vi "CTRE_PigeonIMU_GetAll.vi"(8 "error in (no error)":errorcluster, 11 "PigeonIMUDevRef":T4={"DeviceStatus"={"status"=FALSE, "code"=0, "source"=""}, "Device Number"=0, "Type"=352321536, "Device ID"=0} {"Type" items=["CAN"=352321536, "TalonSRX"=33554432]}) -> (0 "error out":errorcluster, 2 "Get All":T1 {"Calibration"."CurrentMode" items=["BootTareGryoAccel"=0, "Temperature"=1, "Magnetometer12Pt"=2, "Magnetometer360"=3, "Accelerometer"=5]}, 3 "PigeonIMUDevRef":T4={"DeviceStatus"={"status"=FALSE, "code"=0, "source"=""}, "Device Number"=0, "Type"=352321536, "Device ID"=0} {"Type" items=["CAN"=352321536, "TalonSRX"=33554432]})   [LabVIEW 2016]
uses:
  <vilib>/Rock Robotics/WPI/ThirdParty/Sensors/Pigeon IMU/CTRE_PigeonIMU_DeviceRef.ctl
  <vilib>/Rock Robotics/WPI/ThirdParty/Sensors/Pigeon IMU/CTRE_PigeonIMU_ConnectionType.ctl
  <vilib>/Rock Robotics/WPI/ThirdParty/Sensors/Pigeon IMU/CTRE_PigeonIMU_GlobalStatus.ctl
  <vilib>/Rock Robotics/WPI/ThirdParty/Sensors/Pigeon IMU/CTRE_PigeonIMU_PigeonState.ctl
  <vilib>/Rock Robotics/WPI/ThirdParty/Sensors/Pigeon IMU/CTRE_PigeonIMU_CalibrationMode.ctl
  <vilib>/Rock Robotics/WPI/ThirdParty/Sensors/Pigeon IMU/CTRE_PigeonIMU_GlobalOps.ctl
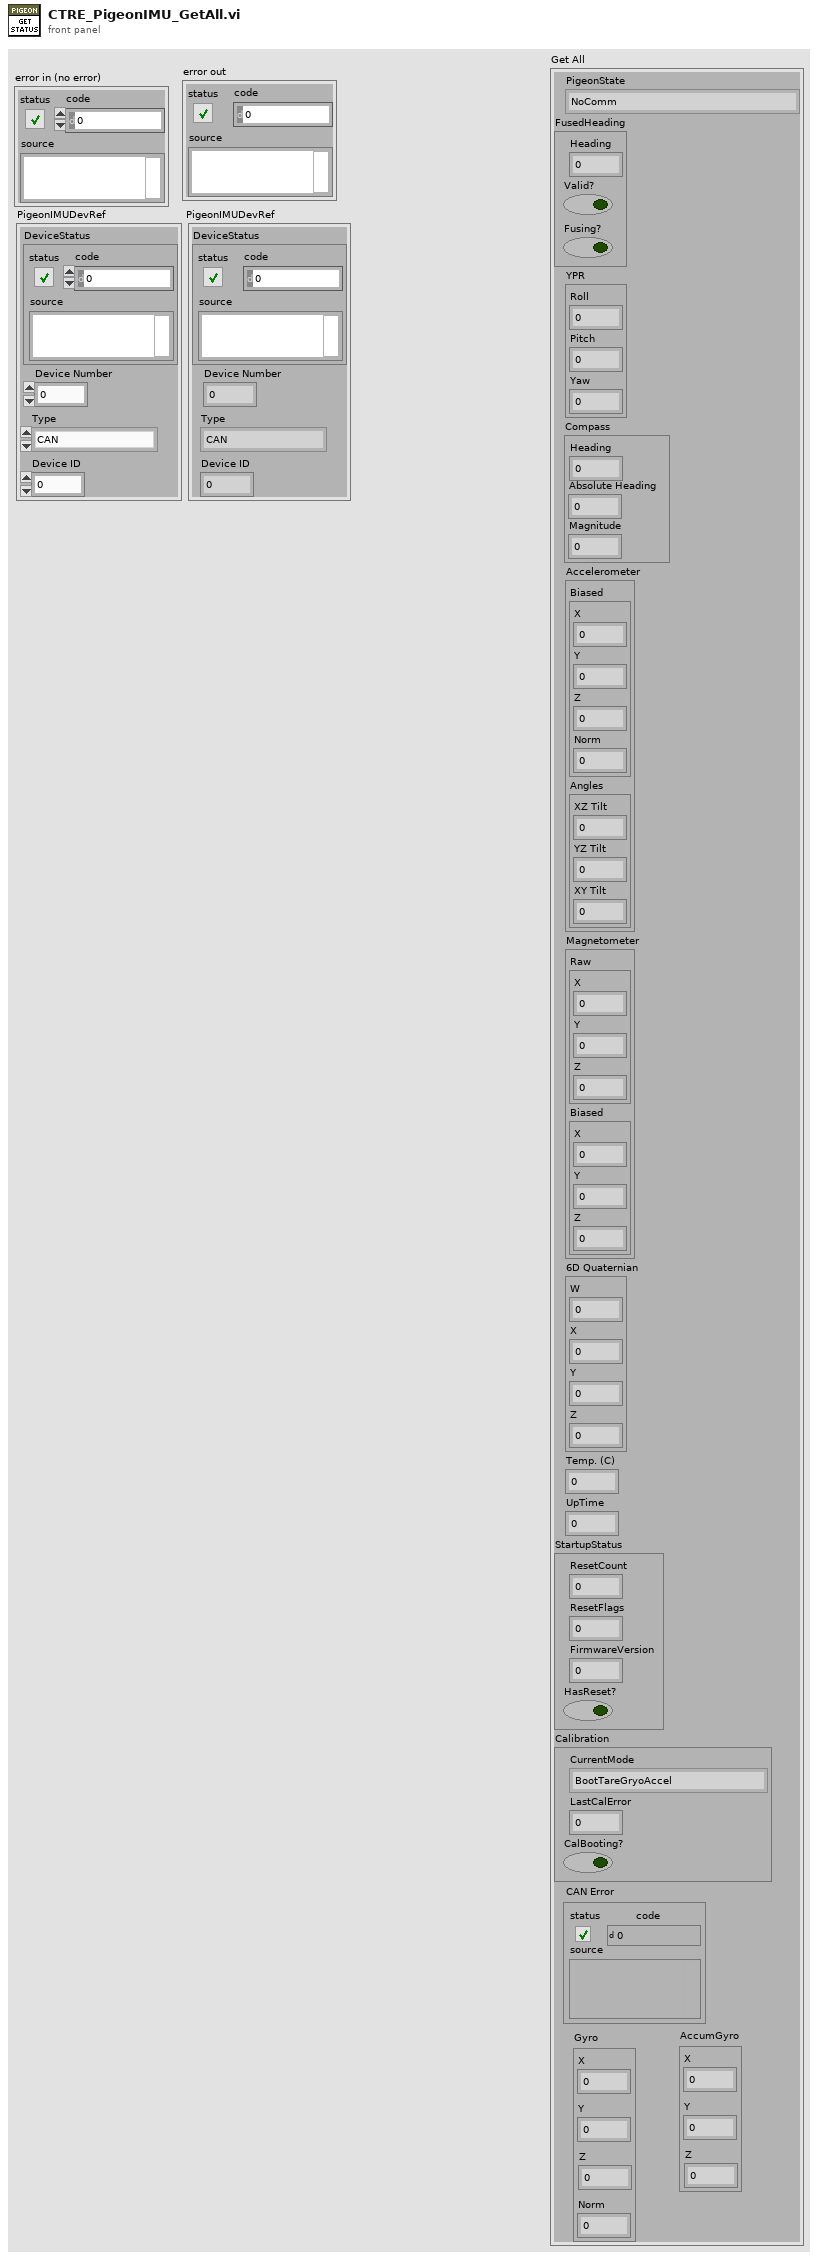
[diagram p1: front panel]
types:
  T1 = typedef "CTRE_PigeonIMU_GlobalStatus.ctl" = cluster{"PigeonState":T2, "FusedHeading":cluster{"Heading":dbl, "Valid?":bool, "Fusing?":bool}, "YPR":cluster{"Yaw":dbl, "Pitch":dbl, "Roll":dbl}, "Compass":cluster{"Heading":dbl, "Magnitude":dbl, "Absolute Heading":dbl}, "Accelerometer":cluster{"Biased":cluster{"X":i16, "Y":i16, "Z":i16, "Norm":i16}, "Angles":cluster{"XZ Tilt":dbl, "YZ Tilt":dbl, "XY Tilt":dbl}}, "Magnetometer":cluster{"Raw":cluster{"X":i16, "Y":i16, "Z":i16}, "Biased":cluster{"X":i16, "Y":i16, "Z":i16}}, "Gyro":cluster{"X":dbl, "Y":dbl, "Z":dbl, "Norm":dbl}, "6D Quaternian":cluster{"W":dbl, "X":dbl, "Y":dbl, "Z":dbl}, "Temp. (C)":dbl, "UpTime":u32, "StartupStatus":cluster{"ResetCount":i32, "ResetFlags":i32, "FirmwareVersion":i32, "HasReset?":bool}, "Calibration":cluster{"CurrentMode":T3, "LastCalError":i32, "CalBooting?":bool}, "CAN Error":errorcluster, "AccumGyro":cluster{"X":dbl, "Y":dbl, "Z":dbl}}
  T2 = typedef "CTRE_PigeonIMU_PigeonState.ctl" = enum16{"NoComm", "Initializing", "Ready", "UserCalibration"}
  T3 = typedef "CTRE_PigeonIMU_CalibrationMode.ctl" = u16
  T4 = typedef "CTRE_PigeonIMU_DeviceRef.ctl" = cluster{"DeviceStatus":errorcluster, "Device Number":u8, "Type":T5, "Device ID":u32}
  T5 = typedef "CTRE_PigeonIMU_ConnectionType.ctl" = u32
  T6 = typedef "CTRE_PigeonIMU_GlobalOps.ctl" = enum16{"Read For Send", "Write Error", "Get All", "Set Control Frame Rate", "Set Enable Frame Rate", "Write After Receive Fused Heading", "Write After Receive YPR", "Write After Receive Status", "Write After Receive Raw Magnetomoter", "Write After Receive Biased Magnetometer", "Write After Receive Biased Accelerometer", "Write After Receive Gyro", "Write After Receive Acceleromter Angles", "Write After Receive Startup Status", "Write After Receive Compass", "Write After Receive Quaternian", "Write After Receive AccumGyro"}
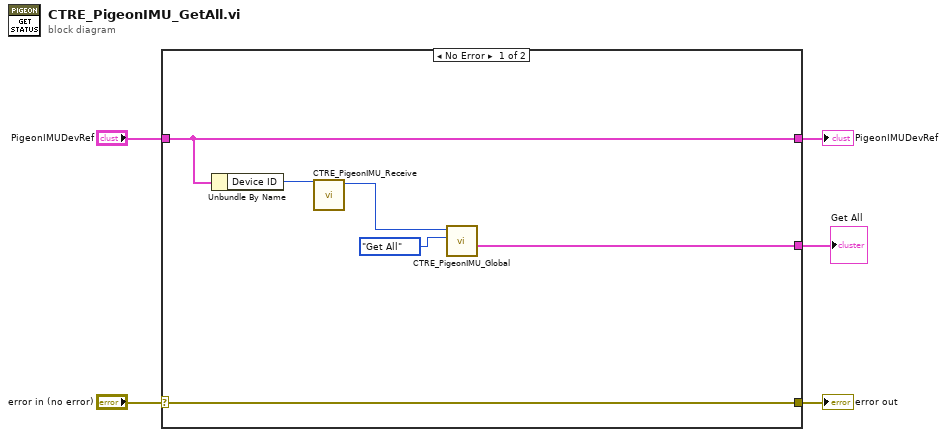
[diagram p0: block diagram]
diagram:
  n1 = case shown="No Error" "error in (no error)" {
    selector: "error in (no error)" -> [w11 w12]
    tunnel: [w11 w12] -> w4
    tunnel: "PigeonIMUDevRef" -> [w10 w13]
    tunnel: [w10 w13] -> w2
    tunnel: [w6 _] -> w1
    frame No Error {
      n2 = Unbundle By Name(w10) -> ("Device ID"=w9:u32)
      n3 = call <vilib>:"CTRE_PigeonIMU_Receive.vi"("Device ID"=w9) -> ("Device ID Out"=w8:u32)  [unwired: 10 in]
      n4 = call <vilib>:"CTRE_PigeonIMU_Global.vi"("Operation"=CTRE_PigeonIMU_GlobalOps."Get All", "Device ID (0)"=w8) -> ("Get All"=w6:T1)  [unwired: 7 in, 2 out]
    }
    frame Error {
    }
  }
  "error out" <- w4
  "PigeonIMUDevRef" <- w2
  "Get All" <- w1
